vi "Global_ACT_Data Out.vi"() -> ()   [LabVIEW 2020, in "Grabber_ACT.lvlib"]
uses:
  Grabber_ACT.lvlib
  <vilib>/Rock Robotics/WPI/ThirdParty/Phoenix-LabVIEW/Motor Controller/Controls/CTRE_Phoenix_MotorControl_ControlMode.ctl
  Shared Code/TypeDefs/Cluster_FX Sensor Values.ctl
  Shared Code/TypeDefs/Cluster_FX CloseLoop Values.ctl
  Shared Code/TypeDefs/Cluster_FX Current Values.ctl
  Shared Code/TypeDefs/Cluster_Grabber HW Outputs.ctl
  Shared Code/TypeDefs/Cluster_Grabber_SW Outputs.ctl
panel:
  in  "ACT_Grabber_SW Output":T1
  out "ACT_Grabber_HW Output":T2
  in  "ACT_Grabber_FX Mode":T6 items=["PercentOutput"=0, "Position"=1, "Velocity"=2, "Current"=3, "Follower"=5, "MotionProfile"=6, "MotionMagic"=7, "MotionProfileArc"=10, "Disabled"=15]
  in  "ACT_Grabber_FX Value":dbl
  in  "ACT_Grabber_CycleTime(S)":dbl
  # "The Names of the Data items in the Global Variable MUST describe who the Single Writer is\nFor Actuator Globals the the naming convention is\n   \nACT_Lib Name_Data Name\n\nExamples:\nACT_Drive_X axis\nACT_Hopper_AgitatorSpeed"
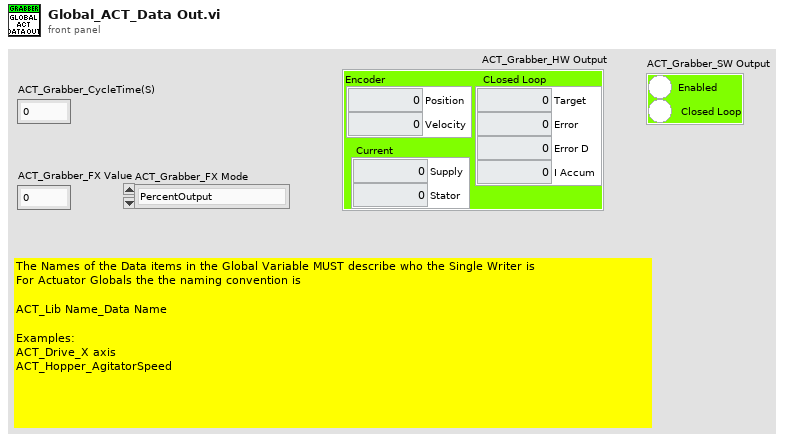
[diagram p1: front panel]
types:
  T1 = typedef "Cluster_Grabber_SW Outputs.ctl" = cluster{"Enabled":bool, "Closed Loop":bool}
  T2 = typedef "Cluster_Grabber HW Outputs.ctl" = cluster{"Encoder":T3, "CLosed Loop":T4, "Current":T5}
  T3 = typedef "Cluster_FX Sensor Values.ctl" = cluster{"Position":i32, "Velocity":i32}
  T4 = typedef "Cluster_FX CloseLoop Values.ctl" = cluster{"Target":dbl, "Error":i32, "Error D":dbl, "I Accum":dbl}
  T5 = typedef "Cluster_FX Current Values.ctl" = cluster{"Supply":dbl, "Stator":dbl}
  T6 = typedef "CTRE_Phoenix_MotorControl_ControlMode.ctl" = u16
diagram:
